vi "SetTriggerAutoReArm.vi"(8 "error in":errorcluster, 10 "TriggerAutoReArm(mSec)":i64, 11 "TriggerBox in":refnum<class "TriggerBox.lvclass">) -> (0 "error out":errorcluster, 3 "TriggerBox out":refnum<class "TriggerBox.lvclass">)   [LabVIEW 2013, in "TriggerBox.lvclass"]
uses:
  TriggerBox.lvclass
  <vilib>/Utility/error.llb/Error Cluster From Error Code.vi
  <vilib>/rvi/errors/niLvFpgaAdjustHostInterfaceError.vi
  <vilib>/rvi/interface/nirviReadWriteControl/nirviReadWriteControl.xnode
  RT/FPGASession/FPGARef.ctl
  FPGA Bitfiles/HWSWTriggerBox_FPGATarget2_TriggerBox_1zhzIx5zPP8.lvbitx
  FPGAMain.vi
  FPGASessionClass/FPGASession.lvclass
  NiFpgaLv.dll
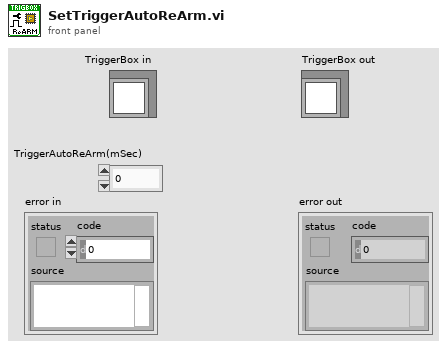
[diagram p1: front panel]
types:
  T1 = typedef "FPGASession.lvclass/FPGARef.ctl" = refnum<k20>
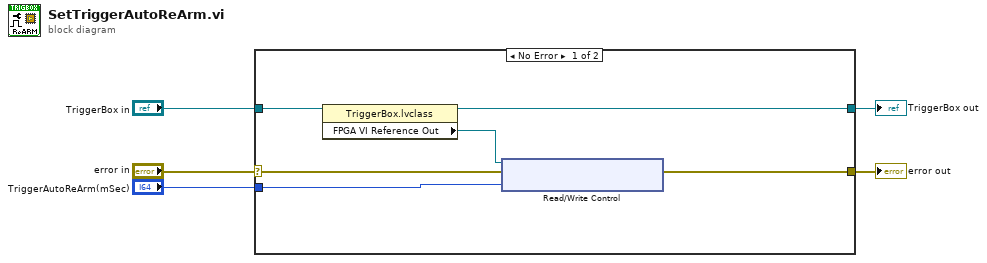
[diagram p0: block diagram]
diagram:
  n1 = case shown="No Error" "error in" {
    selector: "error in" -> [w8 w13]
    tunnel: [w11 w13] -> w2
    tunnel: [w6 w12] -> w3
    tunnel: "TriggerBox in" -> [w9 w12]
    tunnel: "TriggerAutoReArm(mSec)" -> [w10 _]
    frame No Error {
      n2 = property class="TriggerBox.lvclass"(reference=w9) -> (reference out=w6:refnum<class "TriggerBox.lvclass">, "FPGA VI Reference Out"=w7:T1)  [unwired: 1 in, 1 out]
      n3 = xnode "Read/Write Control"("FPGA VI Reference In"=w7, "error in"=w8, "TriggerAutoReArm(mSec)"=w10) -> ("error out"=w11:errorcluster)  [unwired: 1 out]
    }
    frame Error {
    }
  }
  "error out" <- w2
  "TriggerBox out" <- w3
